vi "Autonomous Independent.vi"() -> ()   [LabVIEW 2015]
doc: "This VI is called when autonomous begins, and will automatically be terminated when autonomous ends. You can carry out timed or sensor driven robot movement independently without needing to return to the caller."
uses:
  <vilib>/Rock Robotics/WPI/CAN/TalonSRX/WPI_CANTalonSRX_APIControlMode.ctl
  Robot Global Data.vi
  <vilib>/Rock Robotics/Network Tables/NT Read Numeric Array.vi
  <vilib>/Rock Robotics/Network Tables/NT Read Number.vi
  900/Team900-VIs/Team900SwerveDrive/Team900SwerveDrive.lvlib
panel:
  out "Times: move,     vwait,    vmove,   arm1,     arm2,     close,      lift,        auto+.1, open":dbl[][](array[numeric])
  out "Auto Zone":dbl
  in  "Reverse Pivot Limit":dbl
  in  "Forward Pivot Limit":dbl=512.0
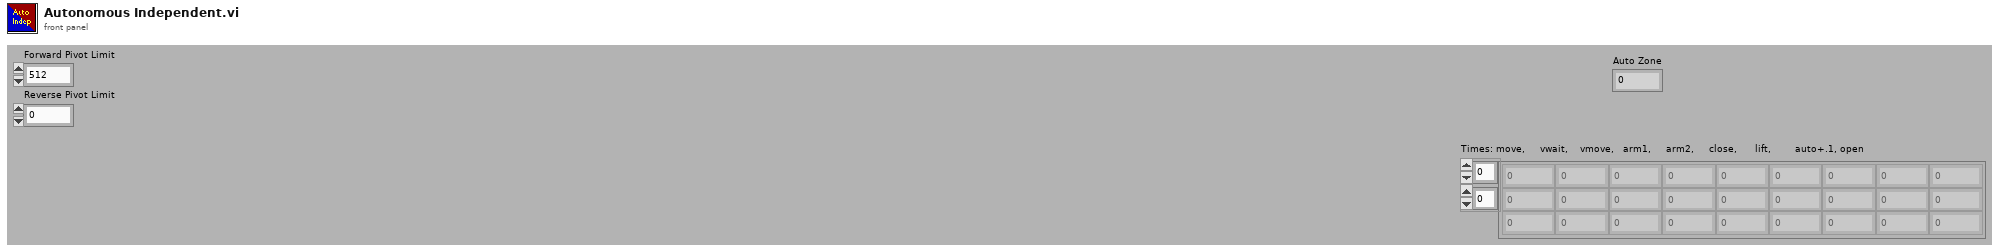
[diagram p1: front panel]
types:
  T1 = typedef "WPI_CANTalonSRX_APIControlMode.ctl" = enum8{"Percent VBus", "Speed", "Position", "Slave", "Unchanged / Invalid"}
  T2 = typedef "WPI_MotorControlDeviceRef.ctl" = cluster{"DeviceStatus":errorcluster, "Type":T3, "PWM":cluster{"PWM Channel":T4, "DeadBand":T5}, "CAN":cluster{"Device Number":u8, "Control Mode":T6, "Semaphore":T7, "Max Vout":dbl, "TalonSRX Control Mode":T1}, "Invert":bool, "TransformRef":T8, "InvTransformRef":T8}
  T3 = typedef "WPI_MotorControlType.ctl" = enum16{"PWM", "CAN", "CANTalonSRX"}
  T4 = typedef "FPGA_DIOPWMChannel.ctl" = enum8{"PWM 0", "PWM 1", "PWM 2", "PWM 3", "PWM 4", "PWM 5", "PWM 6", "PWM 7", "PWM 8", "PWM 9", "PWM MXP 0", "PWM MXP 1", "PWM MXP 2", "PWM MXP 3", "PWM MXP 4", "PWM MXP 5", "PWM MXP 6", "PWM MXP 7", "PWM MXP 8", "PWM MXP 9", "Invalid"}
  T5 = typedef "WPI_PWMDeadband.ctl" = cluster{"Name":string, "maxPositivePwm":i32, "minPositivePwm":i32, "centerPwm":i32, "maxNegativePwm":i32, "minNegativePwm":i32, "angularRange":u16}
  T6 = typedef "WPI_CANJaguar_ControlMode.ctl" = enum8{"Percent VBus", "Current", "Speed", "Position", "Voltage"}
  T7 = typedef "Semaphore RefNum" = refnum<k1>
  T8 = typedef "WPI_PWMTransform_ConPane.ctl" = refnum<vi>
  T9 = cluster{"Extension":enum16{"Go to Setpoint", "Go Past Backward", "Go Past Forward"}, "Pivot":enum16{"Go to Setpoint", "Go Past Backward", "Go Past Forward"}, "Wrist":enum16{"Go to Setpoint", "Go Past Backward", "Go Past Forward"}}
  T10 = typedef "WPI_CANTalonSRX_GlobalStatus.ctl" = cluster{"Applied Throttle":dbl, "Module Enabled":bool, "CAN Error":errorcluster, "Closed Loop Error":dbl, "Forward Limit Switch Closed":bool, "Reverse Limit Switch Closed":bool, "Sensor Position":dbl, "Sensor Velocity":dbl, "Current":dbl, "Sticky Fault - Over Temp":bool, "Sticky Fault - Under Voltage":bool, "Sticky Fault - Forward Limit":bool, "Sticky Fault - Reverse Limit":bool, "Sticky Fault - Forward Soft Limit":bool, "Sticky Fault - Reverse Soft Limit":bool, "Brake is Enabled":bool, "Encoder Position":dbl, "Encoder Velocity":dbl, "Encoder Index Count":dbl, "Encoder A Pin State":bool, "Encoder B Pin State":bool, "Encoder Index Pin State":bool, "Analog In":dbl, "Analog In Velocity":dbl, "Temperature (C)":dbl, "Battery Voltage":dbl}
  T11 = cluster{"proportional gain (Kc)":dbl, "integral time (Ti, min)":dbl, "derivative time (Td, min)":dbl}
  T12 = enum16{"Open", "Close", "Continue", "Stop", "Toggle"}
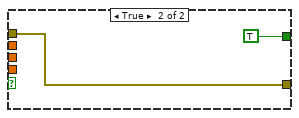
[diagram p3: hidden frame]
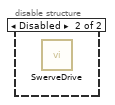
[diagram p5: hidden frame]
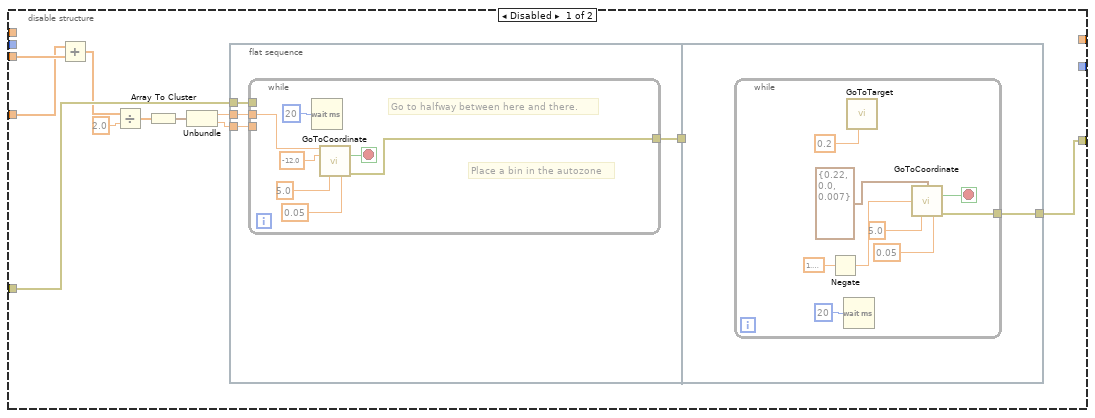
[diagram p7: hidden frame]
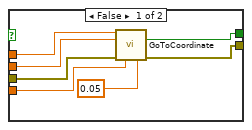
[diagram p8: hidden frame]
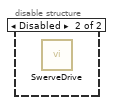
[diagram p13: hidden frame]
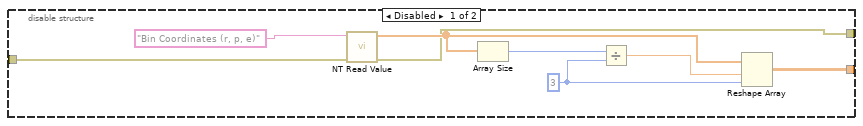
[diagram p14: hidden frame]
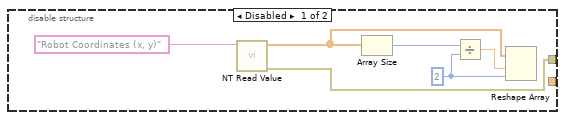
[diagram p15: hidden frame]
diagram:
  w4 = WPI_CANTalonSRX_APIControlMode."Percent VBus" ("Control Mode")
  w19 = TRUE ("Forward Soft Limit Enable")
  w30 = WPI_CANTalonSRX_APIControlMode."Position" ("Control Mode")
  (unwired) "Autonomous sample code is disabled so your robot doesn't unexpectantly run in Autonomous mode.  To enable this code, right-click on the edge of the frame and choose either \"Remove Diagram Disable Structure\" or \"Enable This Subdiagram\". You should only enable one of the samples."
  (unwired) "This function is run in parallel when the autonomous period begins. It will be terminated automatically when the period ends.\n\nNote that all Driver Station inputs are automatically latched and will not change once auto begins."
  # "Every 20ms, report that we are running autonomous\ncode. Loop will abort the same time as the VI."
  # "This gives you the joystick value\nthat is often the throttle"
  # "Use time and/or sensors to control how the robot drives."
  # "This tells you the driver position\nand alliance color"
  n1 = disable-structure shown="Enabled" {
    disable-tunnel: [_ w41] -> w3
    disable-tunnel: [w38 _] -> w31
    frame Disabled {
      w36 = 2 ("dimension size")
      n2 = call-poly <vilib>:"NT Read Value.vi"("Name"="Robot Coordinates (x, y)") -> ("error out"=w38:errorcluster, "Numeric Array"=w34:dbl[])  [unwired: 9 in]
      n3 = Array Size(array=w34) -> (size(s)=w35:i32)
      n4 = Divide(x=w35, y=w36) -> (x/y=w37:dbl)
      n5 = Reshape Array(w34, w37, w36) -> ()  [unwired: 1 out]
    }
    frame Enabled {
      n6 = for {
        N: 6 -> [_]
        tunnel: [w42] -> w41 mode=indexing
        i -> [w48]
        n7 = Number To Decimal String(number=w48) -> (decimal integer string=w46:string)  [unwired: 1 in]
        n8 = Concatenate Strings("RobotX" ("string"), w46) -> (w50:string)
        n9 = Concatenate Strings("RobotY" ("string"), w46) -> (w47:string)
        n10 = call-poly <vilib>:"NT Read Value.vi"("Name"=w50) -> ("Numeric"=w44:dbl)  [unwired: 9 in, 1 out]
        n11 = call-poly <vilib>:"NT Read Value.vi"("Name"=w47) -> ("Numeric"=w43:dbl)  [unwired: 9 in, 1 out]
        n12 = Build Array(w44, w43) -> (w42:dbl[])
      }
    }
  }
  n13 = call <vilib>:"WPI_DriverStationGet Alliance Info.vi"() -> ()  [unwired: 12 out]
  n14 = while {
    stop <- FALSE stop-if-true
    n15 = Wait (ms)(milliseconds to wait=u32 20) -> ()  [unwired: 1 out]
    n16 = call <vilib>:"WPI_DriverStationReport Robot Code State.vi"("Autonomous"=TRUE) -> ()  [unwired: 10 in, 1 out]
  }
  n17 = disable-structure shown="Enabled" {
    disable-tunnel: [w56 w62] -> w33
    disable-tunnel: [w55 w63] -> w32
    disable-tunnel: w31 -> [w54 w63]
    frame Disabled {
      w58 = 3 ("dimension size")
      n18 = call-poly <vilib>:"NT Read Value.vi"("error in"=w54, "Name"="Bin Coordinates (r, p, e)") -> ("error out"=w55:errorcluster, "Numeric Array"=w60:dbl[])  [unwired: 8 in]
      n19 = Array Size(array=w60) -> (size(s)=w59:i32)
      n20 = Divide(x=w59, y=w58) -> (x/y=w57:dbl)
      n21 = Reshape Array(w60, w57, w58) -> (w56:dbl[][])
    }
    frame Enabled {
      n22 = for {
        N: 5 -> [_]
        tunnel: [w70] -> w62 mode=indexing
        i -> [w75]
        n23 = Increment(x=w75) -> (x+1=w65:i32)
        n24 = Number To Decimal String(number=w65) -> (decimal integer string=w66:string)  [unwired: 1 in]
        n25 = Concatenate Strings("RobotR" ("string"), w66) -> (w77:string)
        n26 = Concatenate Strings("RobotP" ("string"), w66) -> (w74:string)
        n27 = Concatenate Strings("RobotE" ("string"), w66) -> (w69:string)
        n28 = call-poly <vilib>:"NT Read Value.vi"("Name"=w77) -> ("Numeric"=w72:dbl)  [unwired: 9 in, 1 out]
        n29 = call-poly <vilib>:"NT Read Value.vi"("Name"=w74) -> ("Numeric"=w71:dbl)  [unwired: 9 in, 1 out]
        n30 = call-poly <vilib>:"NT Read Value.vi"("Name"=w69) -> ("Numeric"=w67:dbl)  [unwired: 9 in, 1 out]
        n31 = Build Array(w72, w71, w67) -> (w70:dbl[])
      }
    }
  }
  n32 = call "ArmGetRefs.vi"() -> ("Wrist Ref"=w13:T2, "Pivot Ref"=w14:T2)  [unwired: 8 in, 2 out]
  n33 = call <vilib>:"WPI_CANTalonSRX_ChangeMode.vi"("Control Mode"=w30, "CAN Talon SRX Ref"=w14) -> ("error out"=w23:errorcluster, "CAN Talon SRX Ref"=w22:T2)  [unwired: 8 in]
  n34 = call <vilib>:"WPI_CANTalonSRX_ChangeMode.vi"("Control Mode"=w30, "CAN Talon SRX Ref"=w13) -> ()  [unwired: 8 in, 2 out]
  n35 = in-place {
    in-place-border: [w80] -> w29
    n36 = call "GoToTarget.vi"("Tolerance Type"=T9 {"Extension"=enum."Go Past Backward", "Pivot"=enum."Go to Setpoint", "Wrist"=enum."Go Past Backward"}, "target wrist angle (rad; relative to ground)"=0.0, "target extension (in.)"=37.5, "target arm angle (rad)"=1.57) -> ("error out"=w80:errorcluster)  [unwired: 4 in, 3 out]
  }
  n37 = call <vilib>:"WPI_CANTalonSRX_GetStatus.vi"("error in (no error)"=w23, "CAN Talon SRX Ref"=w22) -> ("error out"=w26:errorcluster, "Talon SRX Status"=w25:T10, "CAN Talon SRX Ref"=w24:T2)  [unwired: 7 in]
  n38 = Unbundle By Name(w25) -> ("Analog In"=w1:dbl)
  n39 = Add(x=256.0, y=w1) -> (x+y=w9:dbl)
  n40 = global write "Robot Global Data.vi" "Pivot Offset"(w9) -> ()
  n41 = Subtract(x="Forward Pivot Limit", y=w9) -> (x-y=w18:dbl)
  n42 = Subtract(x="Reverse Pivot Limit", y=w9) -> (x-y=w27:dbl)
  n43 = call-poly <vilib>:"NT Read Value.vi"("Name"="Auto Zone") -> ("Numeric"=w8:dbl)  [unwired: 9 in, 1 out]
  "Auto Zone" <- w8
  n44 = call <vilib>:"WPI_CANTalonSRX_ConfigEnabledLimits.vi"("CAN Talon SRX Ref"=w24, "error in (no error)"=w26, "Forward Soft Limit Enable"=w19, "Reverse Soft Limit Enable"=w19) -> ("CAN Talon SRX Ref"=w21:T2, "error out"=w20:errorcluster)  [unwired: 10 in]
  n45 = call <vilib>:"WPI_CANTalonSRX_ConfigSoftLimits.vi"("CAN Talon SRX Ref"=w21, "Forward Limit Position"=w18, "Reverse Limit Position"=w27, "error in (no error)"=w20) -> ("error out"=w2:errorcluster)  [unwired: 10 in, 1 out]
  n46 = call-poly <vilib>:"NT Read Value.vi"("Name"="Auto Type") -> ("Numeric"=w6:dbl)  [unwired: 9 in, 1 out]
  n47 = Bundle(w18, w27) -> (w28:cluster{dbl, dbl})  [unwired: 1 in]
  n48 = global write "Robot Global Data.vi" "Pivot Soft Limits"(w28) -> ()
  n49 = case shown="2" w6 {
    tunnel: w33 -> [w109 _ _ _]
    tunnel: w32 -> [w108 w639 w691 w720]
    tunnel: w29 -> [w111 _ _ _]
    tunnel: w3 -> [w110 _ _ _]
    tunnel: w8 -> [_ _ _ _]
    tunnel: [w107 w638 w691 w720] -> w5
    tunnel: w2 -> [_ _ _ _]
    frame 0, Default {
      # "The one we want to use."
      n50 = flat-sequence {
        tunnel: [w126] -> w106
        tunnel: [w125] -> w105
        tunnel: [w124] -> w104
        tunnel: [w115] -> w103
        tunnel: w109 -> [w126]
        tunnel: w108 -> [w125]
        tunnel: w111 -> [w124]
        tunnel: w110 -> [w116]
        tunnel: [w114] -> w102
        tunnel: [w113] -> w83
        tunnel: w106 -> [w138]
        tunnel: [w138] -> w101
        tunnel: w105 -> [w137]
        tunnel: [w137] -> w99
        tunnel: w104 -> [w136]
        tunnel: [w136] -> w97
        tunnel: w103 -> [w135]
        tunnel: [w135] -> w95
        tunnel: w102 -> [w133]
        tunnel: [w131] -> w93
        tunnel: [w127] -> w84
        tunnel: w83 -> [w127]
        tunnel: w101 -> [w145]
        tunnel: [w145] -> w100
        tunnel: w99 -> [w144]
        tunnel: [w144] -> w98
        tunnel: w97 -> [w143]
        tunnel: [w143] -> w96
        tunnel: w95 -> [w142]
        tunnel: [w142] -> w94
        tunnel: w93 -> [w141]
        tunnel: [w141] -> w92
        tunnel: [w139] -> w85
        tunnel: w84 -> [w139]
        tunnel: [w151] -> w112
        tunnel: w100 -> [w154]
        tunnel: w98 -> [w153]
        tunnel: w96 -> [w152]
        tunnel: w94 -> [w150]
        tunnel: w92 -> [w149]
        tunnel: [w148] -> w91
        tunnel: [w147] -> w90
        tunnel: [w146] -> w86
        tunnel: w85 -> [w146]
        tunnel: w112 -> [w608]
        tunnel: w91 -> [w599]
        tunnel: w90 -> [w598]
        tunnel: [w604] -> w89
        tunnel: [w599] -> w88
        tunnel: [w598] -> w87
        tunnel: w86 -> [w597]
        tunnel: [w637] -> w107
        tunnel: w89 -> [w637]
        tunnel: w88 -> [w629]
        tunnel: w87 -> [w631]
        frame #0 {
          n51 = Delete From Array(array=w116, length=1, index (row)=0) -> (deleted portion=w121:dbl[][], array with subset deleted=w115:dbl[][])  [unwired: 1 in]
          n52 = Index Array(array=w121) -> (element=w117:dbl[])  [unwired: 2 in]
          n53 = Insert Into Array(array=w117, index=2, new element=90.0 ("new element/subarray")) -> (w114:dbl[])
          n54 = Array To Cluster(array=w114) -> (cluster=w122:cluster{"[0]":dbl, "[1]":dbl, "[2]":dbl})
          n55 = global write "Robot Global Data.vi" "Input Coordinates"(w122) -> ()
          n56 = Tick Count (ms)() -> (millisecond timer value=w113:u32)
        }
        frame #1 {
          n57 = Index Array(array=w133) -> (element #1=w130:dbl, element #2=w129:dbl, element #3=w132:dbl)  [unwired: 3 in]
          n58 = global write "Robot Global Data.vi" "Write Coordinates"(TRUE) -> ()
          n59 = expression code="(x/180.0)*pi" "degrees to radians"(w132) -> (w128:dbl)
          n60 = Build Array(w130, w129, w128) -> (w131:dbl[])
        }
        frame #2 {
          n61 = Wait (ms)(milliseconds to wait=u32 100) -> ()  [unwired: 1 out]
        }
        frame #3 {
          # "Sets coordinates to what they should be after moving"
          # "The one we want to use"
          n62 = for {
            tunnel: w150 -> [w231] mode=indexing
            tunnel: w154 -> [w230] mode=indexing
            tunnel: w153 -> [w229]
            tunnel: w152 -> [_]
            tunnel: [w228] -> w151 mode=indexing
            tunnel: w150 -> [w184]
            tunnel: w149 -> [w183]
            tunnel: [w159] -> w147 mode=indexing
            tunnel: [w158] -> w148
            i -> [w192]
            stop <- w190 stop-if-true
            n63 = flat-sequence {
              tunnel: w231 -> [w250]
              tunnel: w230 -> [w252]
              tunnel: [w244] -> w227
              tunnel: [w247] -> w226
              tunnel: [w246] -> w225
              tunnel: w192 -> [w240]
              tunnel: w229 -> [w245]
              tunnel: [w243] -> w224
              tunnel: [w242] -> w223
              tunnel: [w241] -> w222
              tunnel: [w239] -> w221
              tunnel: w183 -> [w237]
              tunnel: [w232] -> w180
              tunnel: w227 -> [w292]
              tunnel: [w292] -> w220
              tunnel: w226 -> [w291]
              tunnel: [w291] -> w219
              tunnel: w225 -> [w290]
              tunnel: [w290] -> w218
              tunnel: [w289] -> w217
              tunnel: w224 -> [w287]
              tunnel: [w287] -> w216
              tunnel: w223 -> [w286]
              tunnel: [w286] -> w215
              tunnel: w222 -> [w288]
              tunnel: [w288] -> w214
              tunnel: w221 -> [w289]
              tunnel: w180 -> [w284]
              tunnel: [w285] -> w179
              tunnel: [w280] -> w178
              tunnel: w220 -> [w317]
              tunnel: [w317] -> w213
              tunnel: w219 -> [w321]
              tunnel: [w322] -> w212
              tunnel: w218 -> [w327]
              tunnel: w217 -> [w326]
              tunnel: [w326] -> w211
              tunnel: w216 -> [w325]
              tunnel: w215 -> [w320]
              tunnel: w214 -> [w324]
              tunnel: [w318] -> w210
              tunnel: [w319] -> w209
              tunnel: [w327] -> w208
              tunnel: w179 -> [w306]
              tunnel: w178 -> [w305]
              tunnel: [w304] -> w177
              tunnel: [w303] -> w176
              tunnel: w213 -> [w366]
              tunnel: w212 -> [w370]
              tunnel: w211 -> [w372]
              tunnel: [w371] -> w207
              tunnel: w210 -> [w369]
              tunnel: [w369] -> w206
              tunnel: [w367] -> w205
              tunnel: w209 -> [w367]
              tunnel: [w370] -> w204
              tunnel: w208 -> [w368]
              tunnel: [w366] -> w203
              tunnel: w177 -> [w361]
              tunnel: w176 -> [w362]
              tunnel: [w360] -> w175
              tunnel: [w359] -> w174
              tunnel: w207 -> [w399]
              tunnel: [w398] -> w202
              tunnel: w206 -> [w402]
              tunnel: [w402] -> w201
              tunnel: w205 -> [w401]
              tunnel: [w401] -> w200
              tunnel: w204 -> [w400]
              tunnel: [w400] -> w199
              tunnel: w203 -> [w397]
              tunnel: w175 -> [w393]
              tunnel: w174 -> [w392]
              tunnel: [w391] -> w173
              tunnel: [w390] -> w172
              tunnel: [w419] -> w198
              tunnel: w202 -> [w420]
              tunnel: w201 -> [w418]
              tunnel: w200 -> [w417]
              tunnel: [w418] -> w197
              tunnel: [w417] -> w196
              tunnel: w199 -> [_]
              tunnel: w173 -> [w413]
              tunnel: w172 -> [w412]
              tunnel: [w410] -> w171
              tunnel: [w411] -> w170
              tunnel: w198 -> [w444]
              tunnel: [w443] -> w188
              tunnel: [w442] -> w187
              tunnel: w197 -> [w442]
              tunnel: [w441] -> w186
              tunnel: w196 -> [w441]
              tunnel: w171 -> [w437]
              tunnel: w170 -> [w436]
              tunnel: [w435] -> w167
              tunnel: [w434] -> w166
              tunnel: w188 -> [w460]
              tunnel: [w460] -> w185
              tunnel: w187 -> [w455]
              tunnel: w186 -> [w456]
              tunnel: [w454] -> w168
              tunnel: w167 -> [w454]
              tunnel: w166 -> [w453]
              tunnel: [w453] -> w165
              tunnel: w185 -> [w464]
              tunnel: [w464] -> w182
              tunnel: [w462] -> w169
              tunnel: w168 -> [w462]
              tunnel: w165 -> [w461]
              tunnel: [w461] -> w164
              tunnel: w182 -> [w468]
              tunnel: [w468] -> w181
              tunnel: w169 -> [w465]
              tunnel: w164 -> [w466]
              tunnel: [w466] -> w163
              tunnel: [w465] -> w162
              tunnel: w181 -> [w481]
              tunnel: w184 -> [w480]
              tunnel: w192 -> [w479]
              tunnel: [w476] -> w195
              tunnel: w190 -> [w473]
              tunnel: [w473] -> w189
              tunnel: w163 -> [w472]
              tunnel: w162 -> [w471]
              tunnel: [w470] -> w161
              tunnel: [w469] -> w160
              tunnel: w195 -> [w576]
              tunnel: w189 -> [w574]
              tunnel: w161 -> [w570]
              tunnel: w160 -> [w569]
              tunnel: [w575] -> w157
              tunnel: [w568] -> w156
              tunnel: [w567] -> w155
              tunnel: [w593] -> w158
              tunnel: [w589] -> w159
              tunnel: [w596] -> w228
              tunnel: w157 -> [w596]
              tunnel: w156 -> [w592]
              tunnel: w155 -> [w590]
              frame #0 {
                n64 = Equal To 0?(x=w240) -> (x = 0?=w233:bool)
                n65 = Array To Cluster(array=w252) -> (cluster=w251:cluster{"[0]":dbl, "[1]":dbl, "[2]":dbl})
                n66 = Unbundle(w251) -> ("[0]"=w248:dbl, "[1]"=w246:dbl, "[2]"=w244:dbl)
                n67 = Insert Into Array(array=w250, index=2, new element=w248) -> (w238:dbl[])
                n68 = Equal?(x=w238, y=w237) -> (x = y?=w236:bool[])
                n69 = And Array Elements(Boolean array=w236) -> (logical AND=w234:bool)
                n70 = And(x=w234, y=w233) -> (x .and. y?=w235:bool)
                n71 = Tick Count (ms)() -> (millisecond timer value=w232:u32)
                n72 = while {
                  tunnel: [w268] -> w247
                  tunnel: w246 -> [_]
                  tunnel: [w253] -> w239
                  tunnel: w245 -> [w255]
                  tunnel: w244 -> [_]
                  tunnel: w238 -> [w266]
                  tunnel: [w265] -> w243
                  tunnel: [w264] -> w242
                  tunnel: [w263] -> w241
                  tunnel: w233 -> [_]
                  tunnel: w235 -> [w254]
                  tunnel: w232 -> [_]
                  stop <- w260 stop-if-true
                  w253 = -0.05 ("target wrist angle (rad; relative to ground)")
                  # "Move in front of bin"
                  n73 = Index Array(array=w266) -> (element #1=w265:dbl, element #2=w264:dbl, element #3=w263:dbl)  [unwired: 3 in]
                  n74 = Wait (ms)(milliseconds to wait=u32 20) -> ()  [unwired: 1 out]
                  n75 = case shown="False" w254 {
                    tunnel: w265 -> [w277 _]
                    tunnel: w264 -> [w276 _]
                    tunnel: w263 -> [w269 _]
                    tunnel: [w275 w278] -> w261
                    tunnel: [w274 TRUE ("Finished")] -> w260
                    tunnel: w255 -> [_ w278]
                    frame False {
                      n76 = call "GoToCoordinate.vi"("Target X"=w277, "Face PID Gains"=T11 {"proportional gain (Kc)"=0.275, "integral time (Ti, min)"=0.0, "derivative time (Td, min)"=0.006}, "Distance PID gains"=T11 {"proportional gain (Kc)"=0.0125, "integral time (Ti, min)"=0.0, "derivative time (Td, min)"=0.00225}, "Target Y"=w276, "Target Angle (rad)"=w269, "Position Tolerance"=5.0, "Angle Tolerance"=0.05) -> ("Finished"=w274:bool, "error out"=w275:errorcluster)  [unwired: 7 in]
                    }
                    frame True {
                    }
                  }
                  n77 = global read "Robot Global Data.vi" "Segment One Length"() -> (w257:dbl)
                  n78 = call "GoToTarget.vi"("Extension Power"=0.3, "Tolerance Type"=T9 {"Extension"=enum."Go to Setpoint", "Pivot"=enum."Go to Setpoint", "Wrist"=enum."Go to Setpoint"}, "error in (no error)"=w255, "target wrist angle (rad; relative to ground)"=w253, "target extension (in.)"=w257, "target arm angle (rad)"=1.0) -> ("error out"=w262:errorcluster)  [unwired: 2 in, 3 out]
                  n79 = Merge Errors(w261, w262) -> (w268:errorcluster)
                }
              }
              frame #1 {
                n80 = Tick Count (ms)() -> (millisecond timer value=w285:u32)
                n81 = while {
                  tunnel: w285 -> [w300]
                  stop <- w296 stop-if-true
                  n82 = Tick Count (ms)() -> (millisecond timer value=w301:u32)
                  n83 = Subtract(x=w301, y=w300) -> (x-y=w299:u32)
                  n84 = Greater?(x=w299, y=u32 1500) -> (0:w297:bool)
                  n85 = call "VisionBinCoordinates.vi"("Minimum Ratio"=0.15, "Vision Array Name"="/VisionTable/VisionArray") -> ("no bin detected"=w293:bool)  [unwired: 2 in, 4 out]
                  n86 = Compound Arithmetic op=OR(invert w293, w297) -> (w296:bool)
                  n87 = Wait (ms)(milliseconds to wait=u32 5) -> ()  [unwired: 1 out]
                  n88 = call "SwerveDriveRotate.vi"() -> ()  [unwired: 17 in, 3 out]
                }
                n89 = Subtract(x=w285, y=w284) -> (x-y=w282:u32)
                n90 = Divide(x=w282, y=1000.0) -> (x/y=w281:dbl)
                n91 = Build Array(w281) -> (w280:dbl[])
              }
              frame #2 {
                # "Turn to face bin based on vision"
                n92 = Cosine(x=w327) -> (cos(x)=w323:dbl)
                n93 = Multiply(x=w323, y=w317) -> (x*y=w314:dbl)
                n94 = call "VisionBinCoordinates.vi"("Distance to Bin"=w314, "Minimum Ratio"=0.15, "Vision Array Name"="/VisionTable/VisionArray") -> ("x Coordinate of Bin"=w313:dbl, "bin angle"=w312:dbl, "no bin detected"=w311:bool)  [unwired: 1 in, 2 out]
                n95 = Not(x=w311) -> (.not. x?=w310:bool)
                n96 = Tick Count (ms)() -> (millisecond timer value=w303:u32)
                n97 = Subtract(x=w303, y=w306) -> (x-y=w308:u32)
                n98 = case shown="True" w310 {
                  tunnel: w325 -> [w328 w339]
                  tunnel: w320 -> [w329 w338]
                  tunnel: w324 -> [_ w341]
                  tunnel: w312 -> [_ w337]
                  tunnel: [w330 w334] -> w322
                  tunnel: w321 -> [w330 w336]
                  tunnel: w313 -> [_ w331]
                  tunnel: [w328 w335] -> w319
                  tunnel: [w329 w338] -> w318
                  tunnel: w303 -> [_ _]
                  frame False {
                  }
                  frame True {
                    n99 = expression code="(x/180.0)*pi" "degrees to radians"(w341) -> (w340:dbl)
                    n100 = global read "Robot Global Data.vi" "Coordinates"() -> (w333:cluster{"X":dbl, "Y":dbl, "Heading":dbl})
                    n101 = Unbundle By Name(w333) -> ("X"=w332:dbl)
                    n102 = disable-structure shown="Enabled" {
                      disable-tunnel: w340 -> [w350 _]
                      disable-tunnel: w339 -> [w343 _]
                      disable-tunnel: w338 -> [_ _]
                      disable-tunnel: w337 -> [w349 _]
                      disable-tunnel: w336 -> [w348 _]
                      disable-tunnel: [w346 _] -> w334
                      disable-tunnel: w331 -> [w345 _]
                      disable-tunnel: [w343 _] -> w335
                      disable-tunnel: w332 -> [w342 _]
                      frame Enabled {
                        n103 = Subtract(x=w350, y=w349) -> (x-y=w347:dbl)
                        n104 = Add(x=w342, y=w345) -> (x+y=w344:dbl)
                        n105 = while {
                          tunnel: w347 -> [_]
                          tunnel: w348 -> [w356]
                          tunnel: [w357] -> w346
                          tunnel: w344 -> [w352]
                          stop <- w358 stop-if-true
                          n106 = Wait (ms)(milliseconds to wait=u32 20) -> ()  [unwired: 1 out]
                          n107 = call "GoToCoordinate.vi"("Target X"=w352, "Distance PID gains"=T11 {"proportional gain (Kc)"=0.0175, "integral time (Ti, min)"=0.0, "derivative time (Td, min)"=0.0001}, "error in (no error)"=w356, "Position Tolerance"=5.0, "Angle Tolerance"=0.05) -> ("Finished"=w358:bool, "error out"=w357:errorcluster)  [unwired: 9 in]
                        }
                      }
                      frame Disabled {
                        n108 = call-poly "SwerveDrive.vi"() -> ()  [unwired: 17 in, 3 out]
                      }
                    }
                  }
                }
                n109 = Divide(x=w308, y=1000.0) -> (x/y=w307:dbl)
                n110 = Build Array (concatenate)(w305, w307) -> (w304:dbl[])
              }
              frame #3 {
                # "Move the arm to the bin"
                n111 = Tick Count (ms)() -> (millisecond timer value=w360:u32)
                n112 = Subtract(x=w360, y=w362) -> (x-y=w364:u32)
                n113 = while {
                  tunnel: w366 -> [w383]
                  tunnel: w370 -> [w389]
                  tunnel: w368 -> [w388]
                  tunnel: w372 -> [w387]
                  tunnel: [w385] -> w371
                  tunnel: w360 -> [_]
                  shift-right: [w378] -> _
                  shift-left: _ -> [w377]
                  shift-left: _ -> [w373]
                  shift-left: _ -> [w376]
                  shift-left: _ -> [w375]
                  shift-left: _ -> [w374]
                  stop <- w379 stop-if-true
                  n114 = global read "Robot Global Data.vi" "Claw Length"() -> (w381:dbl)
                  n115 = Wait (ms)(milliseconds to wait=u32 20) -> ()  [unwired: 1 out]
                  n116 = call-poly "SwerveDrive.vi"() -> ()  [unwired: 17 in, 3 out]
                  n117 = Subtract(x=w383, y=w381) -> (x-y=w382:dbl)
                  n118 = call "GoToTarget.vi"("Extension Power"=0.8, "Tolerance Type"=T9 {"Extension"=enum."Go to Setpoint", "Pivot"=enum."Go to Setpoint", "Wrist"=enum."Go to Setpoint"}, "error in (no error)"=w389, "target wrist angle (rad; relative to ground)"=w387, "target extension (in.)"=w382, "target arm angle (rad)"=w388) -> ("error out"=w385:errorcluster, "finished"=w378:bool)  [unwired: 2 in, 2 out]
                  n119 = Compound Arithmetic op=AND(w378, w377, w376, w375, w374, w373) -> (w379:bool)
                }
                n120 = Divide(x=w364, y=1000.0) -> (x/y=w363:dbl)
                n121 = Build Array (concatenate)(w361, w363) -> (w359:dbl[])
              }
              frame #4 {
                n122 = Tick Count (ms)() -> (millisecond timer value=w390:u32)
                n123 = Subtract(x=w390, y=w393) -> (x-y=w395:u32)
                n124 = while {
                  tunnel: w399 -> [w409]
                  tunnel: [w406] -> w398
                  tunnel: w397 -> [w404]
                  tunnel: w390 -> [_]
                  stop <- w408 stop-if-true
                  n125 = Wait (ms)(milliseconds to wait=u32 20) -> ()  [unwired: 1 out]
                  n126 = call-poly "SwerveDrive.vi"() -> ()  [unwired: 17 in, 3 out]
                  n127 = call "GoToTarget.vi"("Extension Power"=1.0, "Tolerance Type"=T9 {"Extension"=enum."Go Past Forward", "Pivot"=enum."Go to Setpoint", "Wrist"=enum."Go to Setpoint"}, "error in (no error)"=w409, "target extension (in.)"=w404) -> ("error out"=w406:errorcluster, "finished"=w408:bool)  [unwired: 4 in, 2 out]
                }
                n128 = Divide(x=w395, y=1000.0) -> (x/y=w394:dbl)
                n129 = Build Array (concatenate)(w392, w394) -> (w391:dbl[])
              }
              frame #5 {
                n130 = Tick Count (ms)() -> (millisecond timer value=w410:u32)
                n131 = Subtract(x=w410, y=w412) -> (x-y=w415:u32)
                n132 = while {
                  tunnel: w420 -> [w427]
                  tunnel: [w429] -> w419
                  tunnel: w410 -> [_]
                  stop <- w428 stop-if-true
                  n133 = Wait (ms)(milliseconds to wait=u32 20) -> ()  [unwired: 1 out]
                  n134 = call "GoToTarget.vi"("Tolerance Type"=T9 {"Extension"=enum."Go Past Forward", "Pivot"=enum."Go Past Backward", "Wrist"=enum."Go to Setpoint"}, "error in (no error)"=w427) -> ("error out"=w426:errorcluster, "finished"=w425:bool)  [unwired: 6 in, 2 out]
                  n135 = call <vilib>:"WPI_MotorControlRefNum Registry Get.vi"("error in (no error)"=w426, "refnum name"="Claw") -> ("error out"=w432:errorcluster, "MotorControlDevRef"=w430:T2)  [unwired: 8 in]
                  n136 = Select(t=T12."Close" ("Operation"), s=w425, f=T12."Open") -> (s? t:f=w423:T12)
                  n137 = call "Claw Control.vi"("error in (no error)"=w432, "Operation"=w423, "MotorControlDevRef"=w430) -> ("error out"=w429:errorcluster, "Holding"=w428:bool)  [unwired: 3 in, 2 out]
                }
                n138 = Divide(x=w415, y=1000.0) -> (x/y=w414:dbl)
                n139 = Build Array (concatenate)(w413, w414) -> (w411:dbl[])
              }
              frame #6 {
                # "Bring the arm back"
                n140 = Tick Count (ms)() -> (millisecond timer value=w434:u32)
                n141 = Subtract(x=w434, y=w437) -> (x-y=w439:u32)
                n142 = while {
                  tunnel: w444 -> [w452]
                  tunnel: [w449] -> w443
                  tunnel: w434 -> [_]
                  stop <- w451 stop-if-true
                  n143 = global read "Robot Global Data.vi" "Segment One Length"() -> (w445:dbl)
                  n144 = Wait (ms)(milliseconds to wait=u32 20) -> ()  [unwired: 1 out]
                  n145 = call "GoToTarget.vi"("Extension Power"=1.0, "Tolerance Type"=T9 {"Extension"=enum."Go to Setpoint", "Pivot"=enum."Go Past Forward", "Wrist"=enum."Go to Setpoint"}, "error in (no error)"=w452, "target extension (in.)"=w445, "target arm angle (rad)"=0.6) -> ("error out"=w449:errorcluster, "finished"=w451:bool)  [unwired: 3 in, 2 out]
                }
                n146 = Divide(x=w439, y=1000.0) -> (x/y=w438:dbl)
                n147 = Build Array (concatenate)(w436, w438) -> (w435:dbl[])
              }
              frame #7 {
                n148 = global read "Robot Global Data.vi" "Coordinates"() -> (w457:cluster{"X":dbl, "Y":dbl, "Heading":dbl})
                n149 = Unbundle(w457) -> ("Heading"=w458:dbl)  [unwired: 2 out]
                n150 = Bundle(cluster=w457, "X"=w456, "Y"=w455, "Heading"=w458) -> (w459:cluster{"X":dbl, "Y":dbl, "Heading":dbl})
                n151 = global write "Robot Global Data.vi" "Input Coordinates"(w459) -> ()
              }
              frame #8 {
                n152 = global write "Robot Global Data.vi" "Write Coordinates"(TRUE) -> ()
              }
              frame #9 {
                n153 = Wait (ms)(milliseconds to wait=u32 100) -> ()  [unwired: 1 out]
              }
              frame #10 {
                n154 = local read "Auto Zone"() -> (w477:dbl)
                n155 = Greater?(x=w477, y=0.0) -> (0:w474:bool)
                n156 = Compound Arithmetic op=AND(w474, invert w473) -> (w475:bool)
                n157 = case shown="True" w475 {
                  tunnel: w481 -> [w484 w497]
                  tunnel: [w484 w490] -> w476
                  tunnel: w477 -> [_ w496]
                  tunnel: w480 -> [_ w492]
                  tunnel: w479 -> [_ w491]
                  tunnel: w472 -> [w483 w488]
                  tunnel: w471 -> [w482 w487]
                  tunnel: [w483 w486] -> w470
                  tunnel: [w482 w485] -> w469
                  frame False {
                  }
                  frame True {
                    n158 = Increment(x=w491) -> (x+1=w493:i32)
                    n159 = Decrement(x=w496) -> (x-1=w489:dbl)
                    n160 = Index Array(array=w492, index (row)=w491) -> (element=w495:dbl[])  [unwired: 1 in]
                    n161 = Index Array(array=w492, index (row)=w493) -> (element=w494:dbl[])  [unwired: 1 in]
                    n162 = local write "Auto Zone"(w489) -> ()
                    n163 = disable-structure shown="Enabled" {
                      disable-tunnel: w497 -> [w507 w542]
                      disable-tunnel: w495 -> [w504 _]
                      disable-tunnel: w494 -> [w503 w539]
                      disable-tunnel: [w498 w541] -> w490
                      disable-tunnel: w488 -> [_ w533]
                      disable-tunnel: w487 -> [_ w532]
                      disable-tunnel: [_ w531] -> w486
                      disable-tunnel: [_ w530] -> w485
                      frame Disabled {
                        n164 = Add(x=w503, y=w504) -> (x+y=w505:dbl[])
                        n165 = Divide(x=w505, y=2.0) -> (x/y=w502:dbl[])
                        n166 = Array To Cluster(array=w502) -> (cluster=w501:cluster{"[0]":dbl, "[1]":dbl})
                        n167 = Unbundle(w501) -> ("[0]"=w500:dbl, "[1]"=w499:dbl)
                        n168 = flat-sequence {
                          tunnel: w507 -> [w512]
                          tunnel: w500 -> [w511]
                          tunnel: w499 -> [w510]
                          tunnel: [w509] -> w508
                          tunnel: w508 -> [_]
                          tunnel: [w520] -> w498
                          frame #0 {
                            n169 = while {
                              tunnel: w512 -> [_]
                              tunnel: w511 -> [w516]
                              tunnel: w510 -> [_]
                              tunnel: [w514] -> w509
                              stop <- w515 stop-if-true
                              # "Place a bin in the autozone"
                              # "Go to halfway between here and there."
                              n170 = Wait (ms)(milliseconds to wait=u32 20) -> ()  [unwired: 1 out]
                              n171 = call "GoToCoordinate.vi"("Target X"=w516, "Target Y"=-12.0, "Position Tolerance"=5.0, "Angle Tolerance"=0.05) -> ("Finished"=w515:bool, "error out"=w514:errorcluster)  [unwired: 10 in]
                            }
                          }
                          frame #1 {
                            n172 = while {
                              tunnel: [w523] -> w520
                              stop <- w524 stop-if-true
                              n173 = Negate(x=1.5707963267948966) -> (-x=w525:dbl)
                              n174 = Wait (ms)(milliseconds to wait=u32 20) -> ()  [unwired: 1 out]
                              n175 = call "GoToTarget.vi"("Extension Power"=0.2) -> ()  [unwired: 7 in, 4 out]
                              n176 = call "GoToCoordinate.vi"("Face PID Gains"=T11 {"proportional gain (Kc)"=0.22, "integral time (Ti, min)"=0.0, "derivative time (Td, min)"=0.007}, "Target Angle (rad)"=w525, "Position Tolerance"=5.0, "Angle Tolerance"=0.05) -> ("Finished"=w524:bool, "error out"=w523:errorcluster)  [unwired: 10 in]
                            }
                          }
                        }
                      }
                      frame Enabled {
                        n177 = Tick Count (ms)() -> (millisecond timer value=w531:u32)
                        n178 = Index Array(array=w539) -> (element #1=w538:dbl, element #2=w537:dbl)  [unwired: 2 in]
                        n179 = while {
                          tunnel: [w555] -> w543
                          tunnel: w542 -> [w553]
                          tunnel: [w552] -> w540
                          tunnel: w538 -> [w551]
                          tunnel: w537 -> [w550]
                          shift-right: [w549] -> _
                          shift-left: _ -> [_]
                          tunnel: w531 -> [_]
                          stop <- w556 stop-if-true
                          n180 = Wait (ms)(milliseconds to wait=u32 20) -> ()  [unwired: 1 out]
                          n181 = case shown="True" TRUE {
                            tunnel: 5.0 ("Position Tolerance") -> [w564 _]
                            tunnel: w553 -> [w562 w565]
                            tunnel: [w561 w565] -> w552
                            tunnel: w551 -> [w560 _]
                            tunnel: w550 -> [w559 _]
                            tunnel: [w558 TRUE ("Finished")] -> w549
                            frame False {
                              n182 = call "GoToCoordinate.vi"("Target X"=w560, "Target Y"=w559, "error in (no error)"=w562, "Position Tolerance"=w564, "Angle Tolerance"=0.05) -> ("Finished"=w558:bool, "error out"=w561:errorcluster)  [unwired: 9 in]
                            }
                            frame True {
                              n183 = call "SwerveDriveRotate.vi"() -> ()  [unwired: 17 in, 3 out]
                            }
                          }
                          n184 = call "GoToTarget.vi"("Extension Power"=0.8, "Tolerance Type"=T9 {"Extension"=enum."Go to Setpoint", "Pivot"=enum."Go Past Forward", "Wrist"=enum."Go Past Forward"}, "error in (no error)"=w553, "target wrist angle (rad; relative to ground)"=3.141592653589793, "target arm angle (rad)"=3.0) -> ("error out"=w555:errorcluster, "finished"=w556:bool)  [unwired: 3 in, 2 out]
                        }
                        n185 = Subtract(x=w531, y=w533) -> (x-y=w535:u32)
                        n186 = Divide(x=w535, y=1000.0) -> (x/y=w534:dbl)
                        n187 = Build Array (concatenate)(w532, w534) -> (w530:dbl[])
                        n188 = Merge Errors(w543, w540) -> (w541:errorcluster)
                      }
                    }
                  }
                }
              }
              frame #11 {
                n189 = Tick Count (ms)() -> (millisecond timer value=w567:u32)
                n190 = Subtract(x=w567, y=w570) -> (x-y=w572:u32)
                n191 = case shown="False" w574 {
                  tunnel: w576 -> [w579 w588]
                  tunnel: [w578 w588] -> w575
                  tunnel: w567 -> [w577 _]
                  frame False {
                    n192 = while {
                      tunnel: w579 -> [w582]
                      tunnel: [w581] -> w578
                      tunnel: w577 -> [_]
                      stop <- w580 stop-if-true
                      n193 = Wait (ms)(milliseconds to wait=u32 20) -> ()  [unwired: 1 out]
                      n194 = call <vilib>:"WPI_MotorControlRefNum Registry Get.vi"("error in (no error)"=w582, "refnum name"="Claw") -> ("error out"=w586:errorcluster, "MotorControlDevRef"=w583:T2)  [unwired: 8 in]
                      n195 = call "Claw Control.vi"("error in (no error)"=w586, "Operation"=T12."Open", "MotorControlDevRef"=w583) -> ("error out"=w581:errorcluster, "Holding Open"=w580:bool)  [unwired: 3 in, 2 out]
                      n196 = call "SwerveDriveRotate.vi"() -> ()  [unwired: 17 in, 3 out]
                    }
                  }
                  frame True {
                  }
                }
                n197 = Divide(x=w572, y=1000.0) -> (x/y=w571:dbl)
                n198 = Build Array (concatenate)(w569, w571) -> (w568:dbl[])
              }
              frame #12 {
                n199 = Tick Count (ms)() -> (millisecond timer value=w593:u32)
                n200 = Subtract(x=w593, y=w590) -> (x-y=w591:u32)
                n201 = Divide(x=w591, y=1000.0) -> (x/y=w594:dbl)
                n202 = Build Array (concatenate)(w592, w594) -> (w589:dbl[])
              }
            }
            n203 = Increment(x=w192) -> (x+1=w191:i32)
            n204 = call-poly <vilib>:"NT Read Value.vi"("Name"="Num Of Bins To Grab") -> ("Numeric"=w193:dbl)  [unwired: 9 in, 1 out]
            n205 = Equal?(x=w191, y=w193) -> (x = y?=w190:bool)
          }
        }
        frame #4 {
          n206 = global read "Robot Global Data.vi" "Coordinates"() -> (w603:cluster{"X":dbl, "Y":dbl, "Heading":dbl})
          n207 = Unbundle By Name(w603) -> ("X"=w602:dbl)
          n208 = Merge Errors(w608) -> (w607:errorcluster)
          n209 = call-poly <vilib>:"NT Read Value.vi"("Name"="Auto Zone Y") -> ("Numeric"=w600:dbl)  [unwired: 9 in, 1 out]
          n210 = while {
            tunnel: w607 -> [w625]
            tunnel: [w624] -> w606
            tunnel: [w623] -> w605
            tunnel: w602 -> [w622]
            tunnel: w600 -> [w621]
            tunnel: w597 -> [w614]
            stop <- w610 stop-if-true
            n211 = call "GoToCoordinate.vi"("Target X"=w622, "Target Y"=w621, "error in (no error)"=w625) -> ("Finished"=w628:bool, "error out"=w624:errorcluster)  [unwired: 11 in]
            n212 = global read "Robot Global Data.vi" "Segment One Length"() -> (w620:dbl)
            n213 = Wait (ms)(milliseconds to wait=u32 20) -> ()  [unwired: 1 out]
            n214 = Tick Count (ms)() -> (millisecond timer value=w615:u32)
            n215 = Subtract(x=w615, y=w614) -> (x-y=w613:u32)
            n216 = call "GoToTarget.vi"("Extension Power"=0.8, "Tolerance Type"=T9 {"Extension"=enum."Go to Setpoint", "Pivot"=enum."Go to Setpoint", "Wrist"=enum."Go to Setpoint"}, "error in (no error)"=w625, "target wrist angle (rad; relative to ground)"=0.5, "target extension (in.)"=w620, "target arm angle (rad)"=2.0) -> ("error out"=w623:errorcluster, "finished"=w627:bool)  [unwired: 2 in, 2 out]
            n217 = And(x=w628, y=w627) -> (x .and. y?=w611:bool)
            n218 = Greater Or Equal?(x=w613, y=u32 15000) -> (x >= y?=w609:bool)
            n219 = Or(x=w609, y=w611) -> (x .or. y?=w610:bool)
          }
          n220 = Merge Errors(w606, w605) -> (w604:errorcluster)
        }
        frame #5 {
          n221 = Tick Count (ms)() -> (millisecond timer value=w630:u32)
          n222 = Subtract(x=w630, y=w629) -> (x-y=w635:u32)
          n223 = Divide(x=w635, y=1000.0) -> (x/y=w634:dbl)
          n224 = Build Array(w634) -> (w633:dbl[])
          n225 = call "SwerveDriveRotate.vi"() -> ()  [unwired: 17 in, 3 out]
          n226 = Build Array (concatenate)(w631, w633) -> (→"Times: move,     vwait,    vmove,   arm1,     arm2,     close,      lift,        auto+.1, open":dbl[][])
        }
      }
    }
    frame 1 {
      # "Knock Bins Over"
      n227 = flat-sequence {
        tunnel: w639 -> [w645]
        tunnel: [w644] -> w643
        tunnel: w643 -> [w662]
        tunnel: [w661] -> w642
        tunnel: w642 -> [w675]
        tunnel: [w674] -> w641
        tunnel: [w673] -> w638
        tunnel: [w685] -> w640
        tunnel: w641 -> [w685]
        tunnel: w640 -> [w686]
        frame #0 {
          n228 = while {
            tunnel: w645 -> [w647]
            tunnel: [w646] -> w644
            stop <- w648 stop-if-true
            n229 = Wait (ms)(milliseconds to wait=u32 20) -> ()  [unwired: 1 out]
            n230 = call "GoToTarget.vi"("Extension Power"=0.8, "error in (no error)"=w647, "target wrist angle (rad; relative to ground)"=0, "target extension (in.)"=70.0, "target arm angle (rad)"=0.1) -> ("error out"=w651:errorcluster, "finished"=w649:bool)  [unwired: 3 in, 2 out]
            n231 = call <vilib>:"WPI_MotorControlRefNum Registry Get.vi"("error in (no error)"=w651, "refnum name"="Claw") -> ("error out"=w655:errorcluster, "MotorControlDevRef"=w652:T2)  [unwired: 8 in]
            n232 = call "Claw Control.vi"("error in (no error)"=w655, "Operation"=T12."Close", "MotorControlDevRef"=w652) -> ("error out"=w646:errorcluster, "Holding"=w650:bool)  [unwired: 3 in, 2 out]
            n233 = And(x=w649, y=w650) -> (x .and. y?=w648:bool)
          }
        }
        frame #1 {
          n234 = while {
            tunnel: w662 -> [w664]
            tunnel: [w663] -> w661
            stop <- w665 stop-if-true
            n235 = Divide(x=3.141592653589793, y=3) -> (x/y=w666:dbl)
            n236 = Wait (ms)(milliseconds to wait=u32 20) -> ()  [unwired: 1 out]
            n237 = call "GoToCoordinate.vi"("Face PID Gains"=T11 {"proportional gain (Kc)"=0.275, "integral time (Ti, min)"=0.0, "derivative time (Td, min)"=0.006}, "Target Angle (rad)"=w666, "error in (no error)"=w664, "Position Tolerance"=5.0, "Angle Tolerance"=0.05) -> ("Finished"=w665:bool, "error out"=w663:errorcluster)  [unwired: 9 in]
          }
        }
        frame #2 {
          n238 = while {
            tunnel: w675 -> [w678]
            tunnel: [w677] -> w674
            tunnel: [w676] -> w673
            stop <- w679 stop-if-true
            w677 = 110
            (unwired) 0.0
            n239 = Wait (ms)(milliseconds to wait=u32 20) -> ()  [unwired: 1 out]
            n240 = call "GoToCoordinate.vi"("Target X"=w677, "Face PID Gains"=T11 {"proportional gain (Kc)"=0.275, "integral time (Ti, min)"=0.0, "derivative time (Td, min)"=0.006}, "error in (no error)"=w678, "Position Tolerance"=5.0, "Angle Tolerance"=0.05) -> ("Finished"=w679:bool, "error out"=w676:errorcluster)  [unwired: 9 in]
          }
        }
        frame #3 {
          n241 = global write "Robot Global Data.vi" "Write Coordinates"(TRUE) -> ()
        }
        frame #4 {
          n242 = global read "Robot Global Data.vi" "Coordinates"() -> (w688:cluster{"X":dbl, "Y":dbl, "Heading":dbl})
          n243 = Unbundle(w688) -> ("Y"=w687:dbl, "Heading"=w689:dbl)  [unwired: 1 out]
          n244 = Bundle(cluster=w688, "X"=w686, "Y"=w687, "Heading"=w689) -> (w690:cluster{"X":dbl, "Y":dbl, "Heading":dbl})
          n245 = global write "Robot Global Data.vi" "Input Coordinates"(w690) -> ()
        }
      }
    }
    frame 2 {
      # "One that works"
      # "Drive Forward"
      n246 = global read "Robot Global Data.vi" "Coordinates"() -> (w693:cluster{"X":dbl, "Y":dbl, "Heading":dbl})
      n247 = Unbundle By Name(w693) -> ("Y"=w692:dbl)
      n248 = flat-sequence {
        tunnel: w692 -> [w694]
        frame #0 {
          n249 = while {
            tunnel: w694 -> [w700]
            stop <- w699 stop-if-true
            n250 = Wait (ms)(milliseconds to wait=u32 20) -> ()  [unwired: 1 out]
            n251 = global read "Robot Global Data.vi" "Coordinates"() -> (w702:cluster{"X":dbl, "Y":dbl, "Heading":dbl})
            n252 = call-poly "SwerveDrive.vi"("Strafe Joystick Axes"=cluster{"Left":dbl, "Right":dbl} {"Left"=0.0, "Right"=-0.75} ("Trigger Axes"), "Strafe Multiplier"=0.5, "FieldCentric? (T)"=TRUE, "Rotation Multiplier"=0.0, "Max Wheel Speed"=20000.0) -> ()  [unwired: 12 in, 3 out]
            n253 = Unbundle By Name(w702) -> ("Y"=w701:dbl)
            n254 = Subtract(x=w701, y=w700) -> (x-y=w698:dbl)
            n255 = Greater?(x=w698, y=120.0 ("x")) -> (0:w699:bool)
          }
        }
        frame #1 {
          n256 = call-poly "SwerveDrive.vi"("Strafe Joystick Axes"=cluster{"Left":dbl, "Right":dbl} {"Left"=0.0, "Right"=0.0} ("Trigger Axes"), "Strafe Multiplier"=0.5, "FieldCentric? (T)"=FALSE, "Rotation Multiplier"=0.0, "Max Wheel Speed"=20000.0) -> ()  [unwired: 12 in, 3 out]
        }
      }
    }
    frame 3 {
      # "Turn to face bin based on vision"
      # "Testing"
      n257 = call "VisionBinCoordinates.vi"("Distance to Bin"=70.0, "Minimum Ratio"=0.15, "Vision Array Name"="/VisionTable/VisionArray") -> ("x Coordinate of Bin"=w717:dbl, "bin angle"=w716:dbl, "no bin detected"=w715:bool)  [unwired: 1 in, 2 out]
      n258 = Not(x=w715) -> (.not. x?=w714:bool)
      n259 = case shown="True" w714 {
        tunnel: w716 -> [_ w728]
        tunnel: [_ w726] -> w712
        tunnel: w717 -> [_ w727]
        frame False {
        }
        frame True {
          n260 = global read "Robot Global Data.vi" "Coordinates"() -> (w725:cluster{"X":dbl, "Y":dbl, "Heading":dbl})
          n261 = Unbundle By Name(w725) -> ("X"=w724:dbl)
          n262 = disable-structure shown="Enabled" {
            disable-tunnel: w728 -> [_ _]
            disable-tunnel: [w732 _] -> w726
            disable-tunnel: w727 -> [w731 _]
            disable-tunnel: w724 -> [w729 _]
            frame Enabled {
              n263 = Add(x=w729, y=w731) -> (x+y=w730:dbl)
              n264 = while {
                tunnel: [w738] -> w732
                tunnel: w730 -> [w734]
                stop <- w739 stop-if-true
                n265 = Wait (ms)(milliseconds to wait=u32 20) -> ()  [unwired: 1 out]
                n266 = call "GoToCoordinate.vi"("Target X"=w734, "Distance PID gains"=T11 {"proportional gain (Kc)"=0.0175, "integral time (Ti, min)"=0.0, "derivative time (Td, min)"=0.0001}, "Position Tolerance"=5.0, "Angle Tolerance"=0.05) -> ("Finished"=w739:bool, "error out"=w738:errorcluster)  [unwired: 10 in]
              }
            }
            frame Disabled {
              n267 = call-poly "SwerveDrive.vi"() -> ()  [unwired: 17 in, 3 out]
            }
          }
        }
      }
      n268 = while {
        tunnel: w712 -> [w722]
        stop <- FALSE stop-if-true
        n269 = call "SwerveDriveRotate.vi"("error in (no error)"=w722) -> ()  [unwired: 16 in, 3 out]
        n270 = Wait (ms)(milliseconds to wait=u32 20) -> ()  [unwired: 1 out]
      }
    }
  }
  n271 = call "ArmGetRefs.vi"() -> ("Extension Ref"=w11:T2, "Pivot Ref"=w12:T2)  [unwired: 8 in, 2 out]
  n272 = call <vilib>:"WPI_CANTalonSRX_ChangeMode.vi"("error in (no error)"=w5, "Control Mode"=w4, "CAN Talon SRX Ref"=w12) -> ()  [unwired: 7 in, 2 out]
  n273 = call <vilib>:"WPI_CANTalonSRX_ChangeMode.vi"("error in (no error)"=w5, "Control Mode"=w4, "CAN Talon SRX Ref"=w11) -> ()  [unwired: 7 in, 2 out]
